vi "peakFinding getMask.vi"(1 "dataArraySize":i32) -> (0 "diffMatrix":T1)   [LabVIEW 2018]
uses:
  <vilib>/Analysis/Matrix/Datatypes/RealMatrix.ctl
  <vilib>/Analysis/Matrix/Numeric/Conversions/Matrix To Array - RM.vi
  <vilib>/Analysis/Matrix/Numeric/Conversions/Array To Matrix - RA2.vi
  <vilib>/Analysis/Matrix/NI_Matrix.lvlib
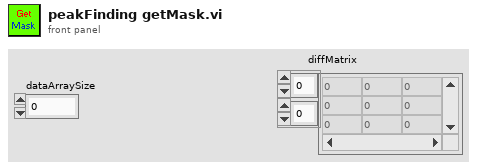
[diagram p1: front panel]
types:
  T1 = typedef "NI_Matrix.lvlib/RealMatrix.ctl" = dbl[][]
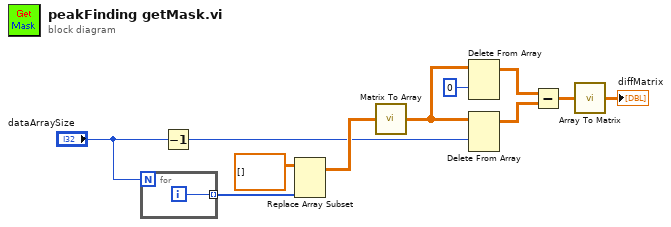
[diagram p0: block diagram]
diagram:
  n1 = for {
    N: "dataArraySize" -> [_]
    tunnel: [w12] -> w10 mode=indexing
    i -> [w12]
  }
  n2 = Decrement(x="dataArraySize") -> (x-1=w5:i32)
  n3 = Replace Array Subset(array=T1 [] ("matrix"), new element=w10) -> (w7:T1)  [unwired: 2 in]
  n4 = call-poly <vilib>:"Matrix To Array.vi"("Real Matrix"=w7) -> ("Real 2D Array"=w8:dbl[][])
  n5 = Delete From Array(array=w8, index (row)=0) -> (array with subset deleted=w4:dbl[][])  [unwired: 2 in, 1 out]
  n6 = Delete From Array(array=w8, index (row)=w5) -> (array with subset deleted=w3:dbl[][])  [unwired: 2 in, 1 out]
  n7 = Subtract(x=w4, y=w3) -> (x-y=w2:dbl[][])
  n8 = call-poly <vilib>:"Array To Matrix.vi"("Real 2D Array"=w2) -> ("Real Matrix"=→"diffMatrix":T1)
